vi "update config.vi"(8 "error in (no error)":errorcluster, 10 "user configurations":T1={"vst_device"=["VST_1", "VST_2"], "RF gain "=10.0, "buffer size"=524288, "center frequency (Hz) "=1000000000.0, "P2P sample rate"=200000000.0, "mode"=enum."5785 - 2*180MHz", "devicess"=["IF_transiver_0", "IF_transiver_1", "IF_transiver_2"], "gen for df"=FALSE, "Rx settings"={"min PW         "=0.0, "max gap        "=0.0, "detection bar"=0.0, "peak detect                        "=FALSE}}, 11 "USRP_1_x_200MHz in":refnum<class "USRP_1_x_200MHz.lvclass">) -> (0 "error out":errorcluster, 1 "min frequency":dbl, 2 "max frequency":dbl, 3 "USRP_1_x_200MHz out":refnum<class "USRP_1_x_200MHz.lvclass">)   [LabVIEW 2021, in "USRP_1_x_200MHz.lvclass"]
uses:
  USRP_1_x_200MHz.lvclass
  <vilib>/userdefined/High Color/nirio_resource_hc.ctl
  USRP_1_x_200MHz.lvclass/USRP_1_x_200MHz.ctl
  pulse_tx_vis/CTL/user config.ctl
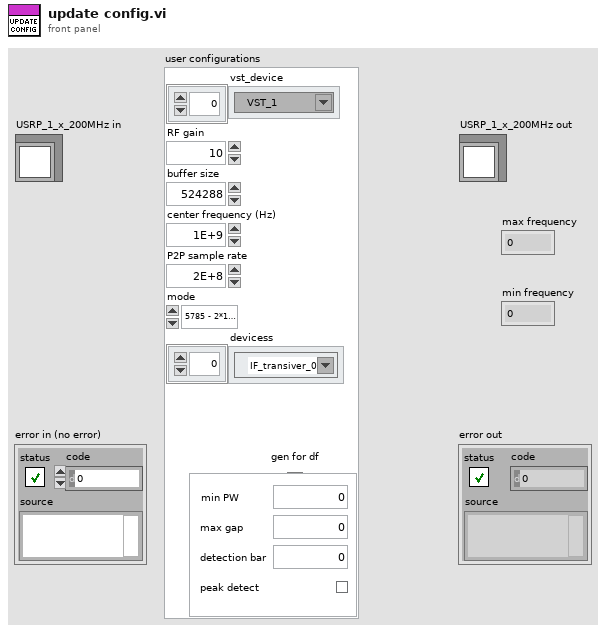
[diagram p1: front panel]
types:
  T1 = typedef "user config.ctl" = cluster{"vst_device":refnum<k15>[], "RF gain ":dbl, "buffer size":u32, "center frequency (Hz) ":dbl, "P2P sample rate":dbl, "mode":enum16{"USRP - 180MHz", "5785 - 2*180MHz", "5785 - 3.2GHz", "P2P - VST"}, "devicess":T2[], "gen for df":bool, "Rx settings":cluster{"min PW         ":dbl, "max gap        ":dbl, "detection bar":dbl, "peak detect                        ":bool}}
  T2 = typedef "nirio_resource_hc.ctl" = tag
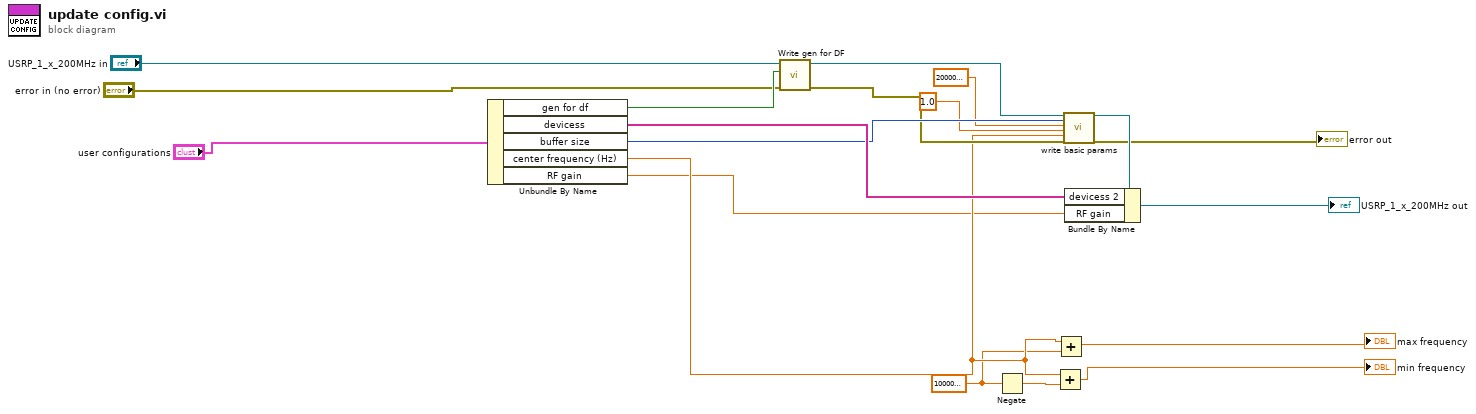
[diagram p0: block diagram]
diagram:
  w9 = 100000000.0 ("Fs  FPGA")
  n1 = Unbundle By Name("user configurations") -> ("gen for df"=w12:bool, "devicess"=w19:T2[], "buffer size"=w17:u32, "center frequency (Hz)"=w10:dbl, "RF gain"=w3:dbl)
  n2 = call-dynamic "Write gen for DF.vi"("error in (no error)"="error in (no error)", "gen for DF"=w12, "device_type in"="USRP_1_x_200MHz in") -> ("error out"=w11:errorcluster, "device_type out"=w13:refnum<class "USRP_1_x_200MHz.lvclass">)  [unwired: 7 in]
  n3 = Negate(x=w9) -> (-x=w18:dbl)
  n4 = Add(x=w10, y=w18) -> (x+y=→"min frequency":dbl)
  n5 = Add(x=w10, y=w9) -> (x+y=→"max frequency":dbl)
  n6 = call-dynamic "write basic params.vi"("device_type in"=w13, "buffer size"=w17, "Fs  FPGA"=200000000.0, "SPC"=1.0 ("Fs  FPGA"), "center frequency (Hz)"=w10, "error in (no error)"=w11) -> ("device_type out"=w14:refnum<class "USRP_1_x_200MHz.lvclass">, "error out"=→"error out":errorcluster)  [unwired: 12 in]
  n7 = Bundle By Name(cluster=w14, "devicess 2"=w19, "RF gain"=w3) -> (→"USRP_1_x_200MHz out":refnum<class "USRP_1_x_200MHz.lvclass">)
